vi "ReportData.vi"() -> ()   [LabVIEW 2023]
uses:
  <vilib>/Utility/NIReport.llb/NI_report.lvclass
  <vilib>/Utility/NIReport.llb/Excel/NI_Excel.lvclass
  <vilib>/Utility/NIReport.llb/Report Type.ctl
  <vilib>/Utility/NIReport.llb/NI_ReportGenerationCore.lvlib
  <vilib>/Utility/NIReport.llb/Append Text Table to Report (wrap).vi
panel:
  in  "stop":bool
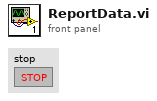
[diagram p1: front panel]
types:
  T1 = typedef "NI_ReportGenerationCore.lvlib/Report Type.ctl" = enum16{"HTML", "Word", "Excel"}
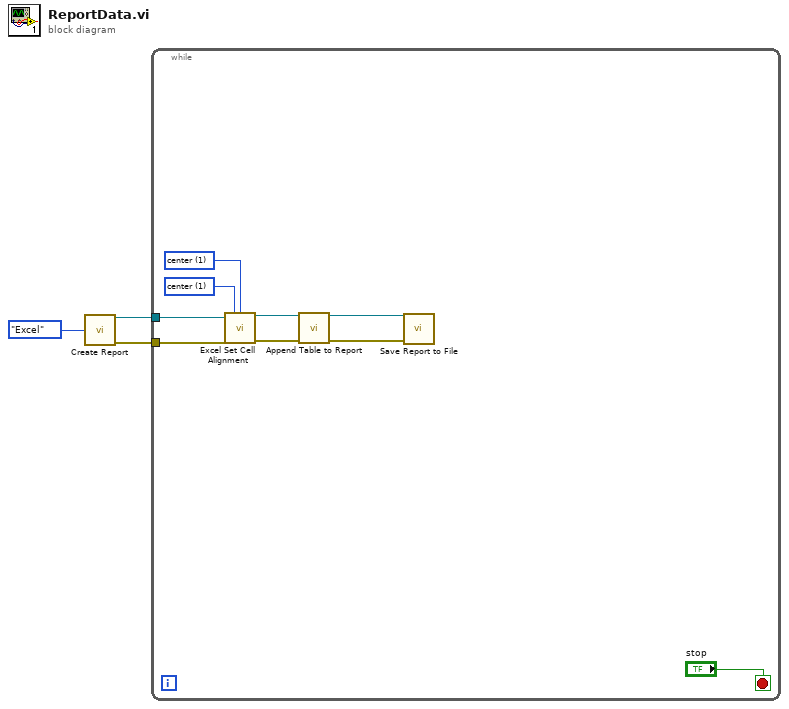
[diagram p0: block diagram]
diagram:
  n1 = call <vilib>:"Create Report.vi"("report type"=Report_Type."Excel") -> ("report out"=w3:refnum<class "NI_report.lvclass">, "error out"=w2:errorcluster)  [unwired: 13 in]
  n2 = while {
    tunnel: w3 -> [w11]
    tunnel: w2 -> [w10]
    stop <- "stop" stop-if-true
    w8 = 1 items=["left", "center", "right"] ("horizontal alignment (left)")
    w9 = 1 items=["top", "center", "bottom"] ("vertical alignment (top)")
    n3 = call <vilib>:"Excel Set Cell Alignment.vi"("report in"=w11, "vertical alignment (top)"=w9, "horizontal alignment (left)"=w8, "error in (no error)"=w10) -> ("report out"=w7:refnum<class "NI_report.lvclass">, "error out"=w6:errorcluster)  [unwired: 10 in]
    n4 = call-poly <vilib>:"Append Table to Report.vi"("report in"=w7, "error in (no error)"=w6) -> ("report out"=w5:refnum<class "NI_report.lvclass">, "error out"=w4:errorcluster)  [unwired: 10 in, 2 out]
    n5 = call-dynamic "Save Report to File.vi"("report in"=w5, "error in (no error)"=w4) -> ()  [unwired: 12 in, 2 out]
  }
